vi "Get Request Type.vi"(8 "error in (no error)":errorcluster, 11 "GetSceneItemTransform in":refnum<class "GetSceneItemTransform.lvclass">) -> (0 "error out":errorcluster, 2 "Request Type":string, 3 "GetSceneItemTransform out":refnum<class "GetSceneItemTransform.lvclass">)   [LabVIEW 2020, in "obs-websocket.lvlib" / "GetSceneItemTransform.lvclass"]
uses:
  GetSceneItemTransform.lvclass
  GetSceneItemTransform.lvclass/GetSceneItemTransform.ctl
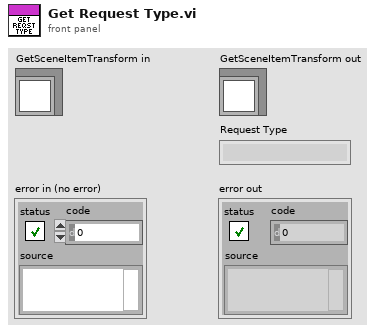
[diagram p1: front panel]
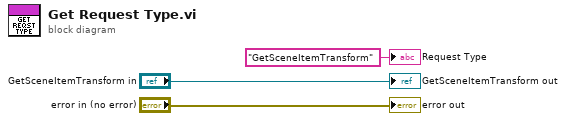
[diagram p0: block diagram]
diagram:
  "error out" <- "error in (no error)"
  "GetSceneItemTransform out" <- "GetSceneItemTransform in"
  "Request Type" <- "GetSceneItemTransform" ("Request Type")
